vi "macro_Pose2d_XYAngleDeg.vi"   [LabVIEW 2019, in "Trajectory_Library.lvlib"]
uses:
  Rotation2d_CreateAngle.vi
  Trajectory_Library.lvlib
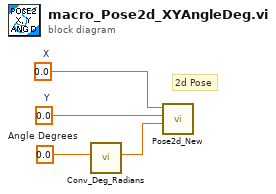
[diagram p0: block diagram]
diagram:
  w1 = 0.0  # X
  w2 = 0.0  # Y
  w4 = 0.0  # Angle Degrees
  # "2d Pose"
  n1 = call "Conv_Deg_Radians.vi"("Degress"=w4) -> ("Radians"=w3:dbl)  [unwired: 10 in]
  n2 = call "Pose2d_New.vi"("Heading"=w3, "Y"=w2, "X"=w1) -> ()  [unwired: 8 in, 1 out]
